vi "Enum Value.vi"(10 "Enumeration":T1) -> (2 "Value":i32)   [LabVIEW 2020, in "AckNackResult.lvlib"]
uses:
  AckNackResult.lvlib
  Enumeration.ctl
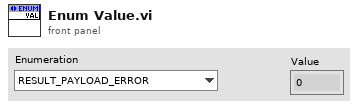
[diagram p1: front panel]
types:
  T1 = typedef "AckNackResult.lvlib/Enumeration.ctl" = enum16{"RESULT_PAYLOAD_ERROR", "RESULT_UNEXPECTED_TYPE", "RESULT_EXPIRED", "RESULT_OUTOFSEQUENCE", "RESULT_DISALLOWED", "RESULT_INVALIDTASK", "RESULT_INVALIDTARGET", "RESULT_UNKNOWN", "RESULT_ACK"}
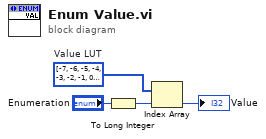
[diagram p0: block diagram]
diagram:
  w4 = i32[] [-7, -6, -5, -4, -3, -2, -1, 0, 1]  # Value LUT
  n1 = To Long Integer(number="Enumeration") -> (32bit integer=w1:i32)
  n2 = Index Array(array=w4, index=w1) -> (element=→"Value":i32)
